vi "Global Load.vi"() -> ()   [LabVIEW 2018]
panel:
  out "K86 True":bool
  out "Flag En Fix4":bool
  out "Flag En Fix3":bool
  out "Flag En Fix2":bool
  out "Flag En Fix1":bool
  out "DUT Fix4":bool
  out "DUT Fix3":bool
  out "DUT Fix2":bool
  out "DUT Fix1":bool
  in  "PRN Fix4":string
  in  "PRN Fix3":string
  in  "PRN Fix2":string
  in  "PRN Fix1":string
  out "Print Fix 4":bool
  out "Print Fix3":bool
  out "Print Fix2":bool
  out "Print Fix1":bool
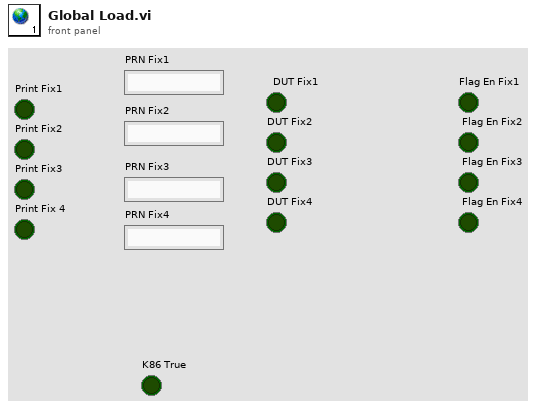
[diagram p1: front panel]
diagram:
